vi "PrimaryInterfaceIsNewDataAvailable.vi"(8 "PrimaryInterface":refnum<k24>, 11 "error in":errorcluster) -> (0 "Data available":bool, 3 "error out":errorcluster)   [LabVIEW 2024, in "UnderAutomation.UniversalRobots.lvlib"]
uses:
  UnderAutomation.UniversalRobots.lvlib
  C:/Users/fg/Documents/UniversalRobots.vi/LabVIEW_2024/UnderAutomation.UniversalRobots/lib/UnderAutomation.UniversalRobots.dll
  lib/UnderAutomation.UniversalRobots.dll
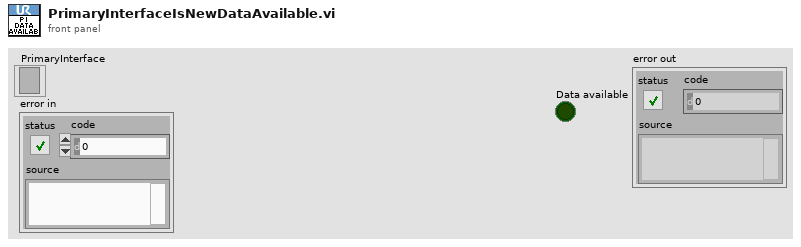
[diagram p1: front panel]
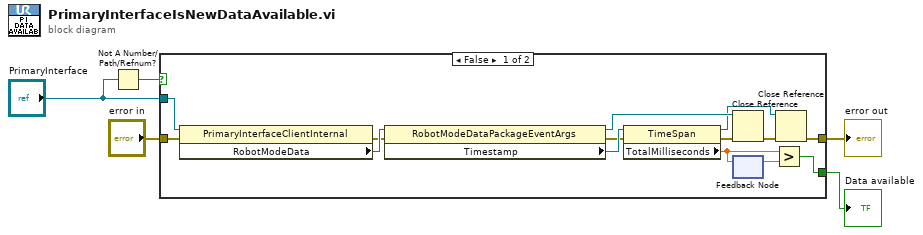
[diagram p0: block diagram]
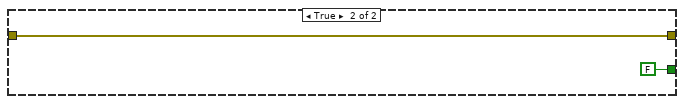
[diagram p2: hidden frame]
diagram:
  n1 = Not A Number/Path/Refnum?(number/path/refnum="PrimaryInterface") -> (NaN/Path/Refnum?=w1:bool)
  n2 = case shown="False" w1 {
    tunnel: "error in" -> [w15 w21]
    tunnel: "PrimaryInterface" -> [w8 _]
    tunnel: [w7 w21] -> w3
    tunnel: [w6 FALSE] -> w2
    frame False {
      n3 = property class="PrimaryInterfaceClientInternal"(reference=w8, error in=w15) -> (error out=w14:errorcluster, "RobotModeData"=w19:refnum<k24>)  [unwired: 1 out]
      n4 = property class="RobotModeDataPackageEventArgs"(reference=w19, error in=w14) -> (reference out=w12:refnum<k24>, error out=w13:errorcluster, "Timestamp"=w18:refnum<k24>)
      n5 = property class="TimeSpan"(reference=w18, error in=w13) -> (reference out=w11:refnum<k24>, error out=w10:errorcluster, "TotalMilliseconds"=w17:dbl)
      n6 = Close Reference(reference=w12, error in (no error)=w10) -> (error out=w9:errorcluster)
      n7 = feedback #1() -> (w16:dbl)  [unwired: 1 in]
      n8 = feedback-in #1(w17) -> ()
      n9 = Greater?(x=w17, y=w16) -> (0:w6:bool)
      n10 = Close Reference(reference=w11, error in (no error)=w9) -> (error out=w7:errorcluster)
    }
    frame True {
    }
  }
  "error out" <- w3
  "Data available" <- w2
